vi "Convert Config.vi"(8 "error in (no error)":errorcluster, 10 "To":refnum<class "Config Storage.lvclass">, 11 "From":refnum<class "Config Storage.lvclass">) -> (0 "error out":errorcluster)   [LabVIEW 2020, in "CDM-Config.lvlib"]
doc: "Converts a saved config file from a source format into a destination format. For example, this can be used to convert a SQLite stored config into JSON for easier viewing/diffing."
uses:
  CDM-Config.lvlib
  Config Storage/Config Storage.lvclass
  Config Manager/Config Manager.lvclass
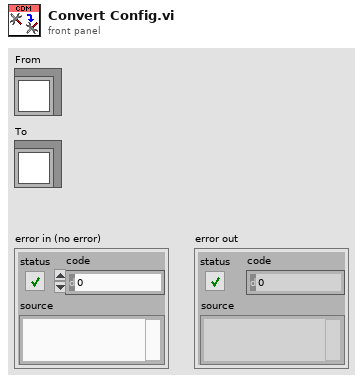
[diagram p1: front panel]
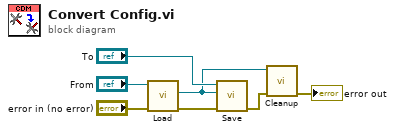
[diagram p0: block diagram]
diagram:
  n1 = call "Load.vi"("error in (no error)"="error in (no error)", "Config Storage in"="From") -> ("error out"=w5:errorcluster, "Config"=w3:refnum<class "Config Manager.lvclass">)  [unwired: 7 in, 1 out]
  n2 = call "Save.vi"("error in (no error)"=w5, "Config"=w3, "Config Storage in"="To") -> ("error out"=w2:errorcluster)  [unwired: 7 in, 1 out]
  n3 = call "Cleanup.vi"("error in (no error)"=w2, "Config Manager in"=w3) -> ("error out"=→"error out":errorcluster)  [unwired: 9 in]
